vi "reset_data_queue.vi"(8 "error in (no error)":errorcluster, 11 "GenericToplevelComponent in":refnum<class "GenericToplevelComponent.lvclass">) -> (0 "error out":errorcluster, 3 "GenericToplevelComponent out":refnum<class "GenericToplevelComponent.lvclass">)   [LabVIEW 2010, in "GenericToplevelComponent.lvclass"]
uses:
  GenericToplevelComponent.lvclass
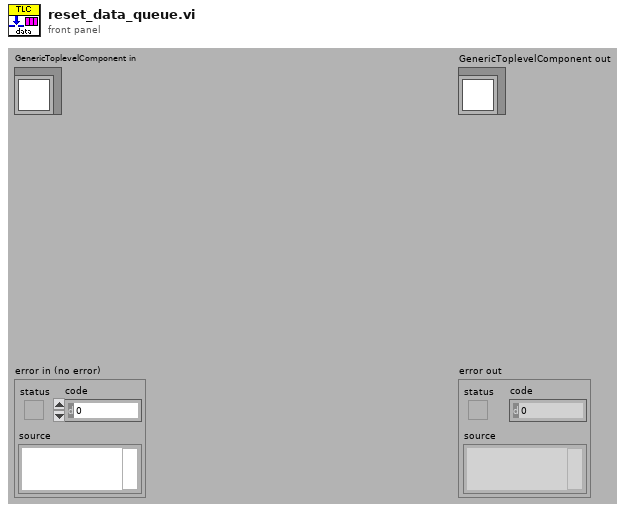
[diagram p1: front panel]
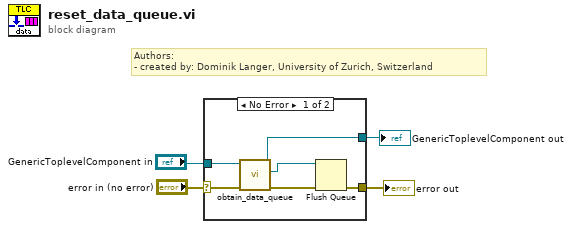
[diagram p0: block diagram]
diagram:
  # "Authors: \n- created by: Dominik Langer, University of Zurich, Switzerland"
  n1 = case shown="No Error" "error in (no error)" {
    selector: "error in (no error)" -> [w9 w12]
    tunnel: [w10 w12] -> w3
    tunnel: [w7 w11] -> w4
    tunnel: "GenericToplevelComponent in" -> [w8 w11]
    frame No Error {
      n2 = call-dynamic "obtain_data_queue.vi"("error in (no error)"=w9, "GenericToplevelComponent in"=w8) -> ("error out"=w5:errorcluster, "data queue"=w6:refnum<queue>, "GenericToplevelComponent out"=w7:refnum<class "GenericToplevelComponent.lvclass">)  [unwired: 7 in]
      n3 = Flush Queue(queue=w6, error in (no error)=w5) -> (error out=w10:errorcluster)  [unwired: 2 out]
    }
    frame Error {
    }
  }
  "error out" <- w3
  "GenericToplevelComponent out" <- w4
